vi "Auto_Routine_BlueRightTwoPieceTRAJ.vi"   [LabVIEW 2023]
uses:
  Shoulder/ShoulderGetSetpointEnum.ctl
  Trajectory/TrajectoryGlobals.vi
  <vilib>/Rock Robotics/WPI/ThirdParty/JAS_Junk/TrajLib/Trajectory_Library.lvlib
types:
  T1 = typedef "ShoulderGetSetpointEnum.ctl" = enum16{"ShoulderRest", "ShoulderSpeaker", "ShoulderAmp"}
  T2 = typedef "ShoulderGetSetpointEnum.ctl" = enum16{"ShoulderRest", "ShoulderShoot", "ShoulderAmp", "ArmFloorPickup", "ArmAmpDeposit", "ArmSpeakerShoot", "ArmStartPosition", "ArmRestPosition", "ArmSourceIntake", "ArmAwayShoot"}
  T3 = typedef "Trajectory_Library.lvlib/TRAJECTORY.ctl" = cluster{"TotalTImeSecs":dbl, "States":T4[]}
  T4 = typedef "Trajectory_Library.lvlib/TRAJ_STATE.ctl" = cluster{"TimeSeconds":dbl, "Velocity":dbl, "Acceleration":dbl, "POSE":T5, "Curvature":dbl}
  T5 = typedef "Trajectory_Library.lvlib/POSE2D.ctl" = cluster{"TRANSLATION":T6, "ROTATION":T7}
  T6 = typedef "Trajectory_Library.lvlib/TRANSLATION2D.ctl" = cluster{"X":dbl, "Y":dbl}
  T7 = typedef "Trajectory_Library.lvlib/ROTATION2D.ctl" = cluster{"VALUE":dbl, "COS":dbl, "SIN":dbl}
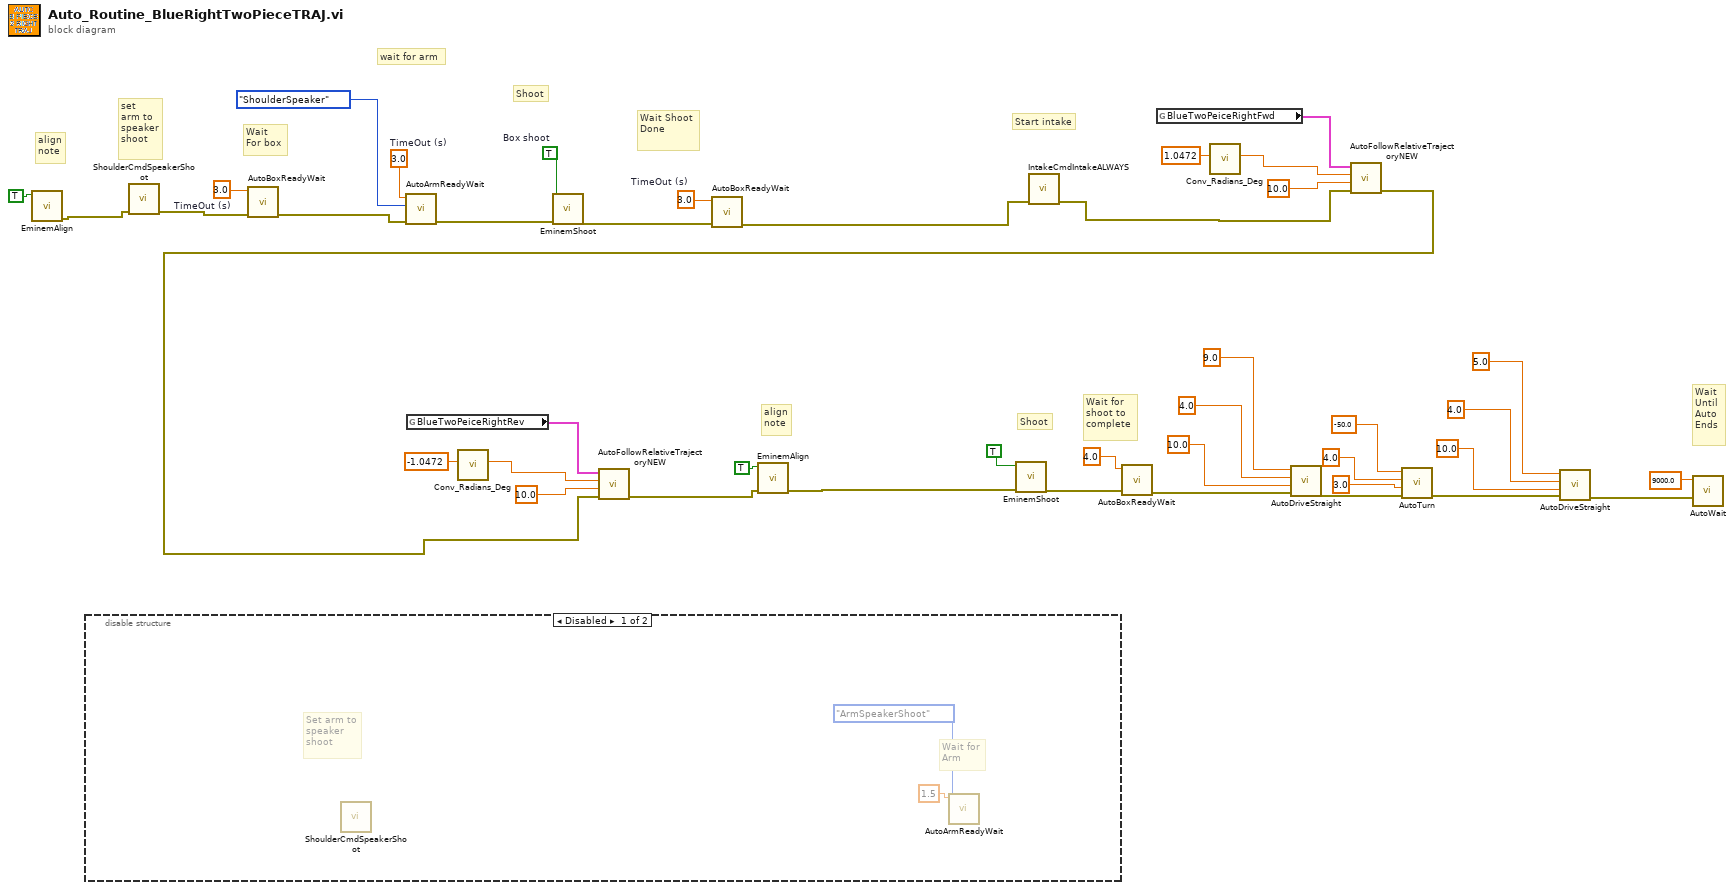
[diagram p0: block diagram]
diagram:
  w35 = 3.0  # TimeOut (s)
  w42 = TRUE  # Box shoot
  w41 = 3.0  # TimeOut (s)
  w38 = 3.0  # TimeOut (s)
  # "align\nnote"
  # "Wait\nUntil\nAuto \nEnds"
  # "Wait for\nshoot to\ncomplete"
  # "Shoot"
  # "Start intake"
  # "Wait Shoot\nDone"
  # "Shoot"
  # "Wait\nFor box"
  # "set \narm to\nspeaker\nshoot"
  # "align\nnote"
  # "wait for arm"
  n1 = call "EminemAlign.vi"("box align"=TRUE) -> ("error out"=w36:errorcluster)  [unwired: 10 in]
  n2 = disable-structure shown="Disabled" {
    frame Disabled {
      # "Wait for\nArm"
      # "Set arm to\nspeaker \nshoot"
      n3 = call "ShoulderCmdSpeakerShoot.vi"() -> ()  [unwired: 11 in, 1 out]
      n4 = call "AutoArmReadyWait.vi"("ArmSetpoints"=ShoulderGetSetpointEnum."ArmSpeakerShoot", "TimeOut (s)"=1.5) -> ("error out"=w44:errorcluster, "error in (no error)"=w43:errorcluster)  [unwired: 8 in]
    }
    frame Enabled {
    }
  }
  n5 = call "ShoulderCmdSpeakerShoot.vi"("error in (no error)"=w36) -> ("error out"=w34:errorcluster)  [unwired: 10 in]
  n6 = call "AutoBoxReadyWait.vi"("error in (no error)"=w34, "TimeOut (s)"=w35) -> ("error out"=w33:errorcluster)  [unwired: 9 in]
  n7 = call "AutoArmReadyWait.vi"("error in (no error)"=w33, "ArmSetpoints"=ShoulderGetSetpointEnum."ShoulderSpeaker", "TimeOut (s)"=w41) -> ("error out"=w39:errorcluster)  [unwired: 8 in]
  n8 = global read "TrajectoryGlobals.vi" "BlueTwoPeiceRightRev"() -> (w24:T3)
  n9 = call <vilib>:"Conv_Radians_Deg.vi"("Radians"=-1.0472) -> ("Degrees"=w22:dbl)  [unwired: 10 in]
  n10 = call "EminemShoot.vi"("error in (no error)"=w39, "Box shoot"=w42) -> ("error out"=w40:errorcluster)  [unwired: 9 in]
  n11 = call "AutoBoxReadyWait.vi"("error in (no error)"=w40, "TimeOut (s)"=w38) -> ("error out"=w2:errorcluster)  [unwired: 9 in]
  n12 = call "IntakeCmdIntakeALWAYS.vi"("error in (no error)"=w2) -> ("error out"=w1:errorcluster)  [unwired: 10 in]
  n13 = global read "TrajectoryGlobals.vi" "BlueTwoPeiceRightFwd"() -> (w32:T3)
  n14 = call <vilib>:"Conv_Radians_Deg.vi"("Radians"=1.0472) -> ("Degrees"=w30:dbl)  [unwired: 10 in]
  n15 = call "AutoFollowRelativeTrajectoryNEW.vi"("error in (no error)"=w1, "TimeOut (s)"=10.0, "End Orientation"=w30, "Trajectory"=w32) -> ("error out"=w5:errorcluster)  [unwired: 7 in]
  n16 = call "AutoFollowRelativeTrajectoryNEW.vi"("error in (no error)"=w5, "TimeOut (s)"=10.0, "End Orientation"=w22, "Trajectory"=w24) -> ("error out"=w15:errorcluster)  [unwired: 7 in]
  n17 = call "EminemAlign.vi"("error in (no error)"=w15, "box align"=TRUE) -> ("error out"=w4:errorcluster)  [unwired: 9 in]
  n18 = call "EminemShoot.vi"("error in (no error)"=w4, "Box shoot"=TRUE) -> ("error out"=w27:errorcluster)  [unwired: 9 in]
  n19 = call "AutoBoxReadyWait.vi"("error in (no error)"=w27, "TimeOut (s)"=4.0) -> ("error out"=w20:errorcluster)  [unwired: 9 in]
  n20 = call "AutoDriveStraight.vi"("error in (no error)"=w20, "TimeOut (s)"=10.0, "MaxSpeed (ft/s)"=4.0, "Dist (ft)"=9.0) -> ("error out"=w9:errorcluster)  [unwired: 7 in]
  n21 = call "AutoTurn.vi"("error in (no error)"=w9, "TimeOut (s)"=3.0, "MaxSpeed (ft/s)"=4.0, "degrees"=-50.0) -> ("error out"=w11:errorcluster)  [unwired: 7 in]
  n22 = call "AutoDriveStraight.vi"("error in (no error)"=w11, "TimeOut (s)"=10.0, "MaxSpeed (ft/s)"=4.0, "Dist (ft)"=5.0) -> ("error out"=w10:errorcluster)  [unwired: 7 in]
  n23 = call "AutoWait.vi"("error in (no error)"=w10, "TimeOut (s)"=9000.0) -> ()  [unwired: 9 in, 1 out]
